vi "niRFUtil WFM Remove Gain Imbalance - Coarse.vi"(0 "Descrambled Chips In":T1 {"y" format="%.2f"; "dx" format="%^.2e"; "x0" format="%^.2e"}) -> (2 "Corrected Descrambled Chips Out":T1 {"y" format="%.2f"; "dx" format="%^.2e"; "x0" format="%^.2e"}, 3 "Gain Imbalance (dB)":sgl format="%.2f")   [LabVIEW 2015, in "niRFUtil.lvlib"]
doc: "(c) Copyright 2006, National Instruments, Inc. This VI may not be duplicated, sold, or distributed without written consent from National Instruments."
uses:
  niRFUtil.lvlib
  Includes/niRFUtil INC Complex Waveform.ctl
  Includes/niRFUtil INC Complex Array.ctl
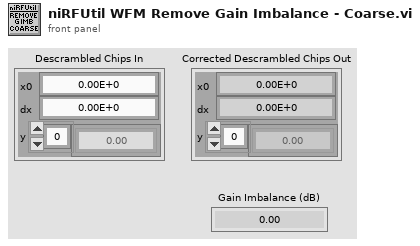
[diagram p1: front panel]
types:
  T1 = typedef "niRFUtil.lvlib/niRFUtil INC Complex Waveform.ctl" = cluster{"x0":dbl, "dx":dbl, "y":T2}
  T2 = typedef "niRFUtil.lvlib/niRFUtil INC Complex Array.ctl" = csg[]
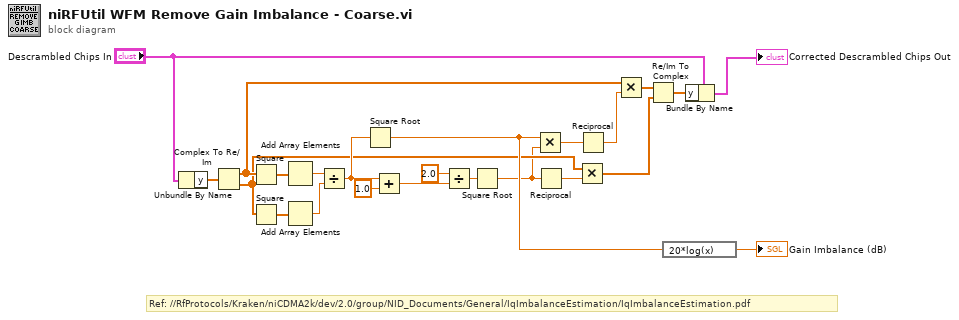
[diagram p0: block diagram]
diagram:
  # "Ref: //RfProtocols/Kraken/niCDMA2k/dev/2.0/group/NID_Documents/General/IqImbalanceEstimation/IqImbalanceEstimation.pdf"
  n1 = Unbundle By Name("Descrambled Chips In") -> ("y"=w23:T2)
  n2 = Complex To Re/Im(x + iy=w23) -> (x=w12:sgl[], y=w10:sgl[])
  n3 = Square(x=w12) -> (x^2=w22:sgl[])
  n4 = Square(x=w10) -> (x^2=w21:sgl[])
  n5 = Add Array Elements(numeric array=w22) -> (sum=w20:sgl)
  n6 = Add Array Elements(numeric array=w21) -> (sum=w19:sgl)
  n7 = Divide(x=w20, y=w19) -> (x/y=w18:sgl)
  n8 = Square Root(x=w18) -> (sqrt(x)=w13:sgl)
  n9 = Add(x=w18, y=sgl 1.0) -> (x+y=w16:sgl)
  n10 = Divide(x=sgl 2.0, y=w16) -> (x/y=w14:sgl)
  n11 = Square Root(x=w14) -> (sqrt(x)=w9:sgl)
  n12 = Multiply(x=w13, y=w9) -> (x*y=w11:sgl)
  n13 = Reciprocal(x=w9) -> (1/x=w2:sgl)
  n14 = Multiply(x=w10, y=w2) -> (x*y=w7:sgl[])
  n15 = Reciprocal(x=w11) -> (1/x=w3:sgl)
  n16 = Multiply(x=w12, y=w3) -> (x*y=w8:sgl[])
  n17 = Re/Im To Complex(1:w7, 2:w8) -> (0:w6:csg[])
  n18 = expression code="20*log(x)"(w13) -> (→"Gain Imbalance (dB)":sgl)
  n19 = Bundle By Name(cluster="Descrambled Chips In", "y"=w6) -> (→"Corrected Descrambled Chips Out":T1)
